vi "Periodic Tasks.vi"(8 "error in":errorcluster) -> ()   [LabVIEW 2017]
doc: "This VI runs in parallel to other robot code. It can contain as many user-defined periodic loops as you need. These can carry out PID or other sorts of timed response."
uses:
  <vilib>/Rock Robotics/Network Tables/NT Write Number.vi
  <vilib>/Rock Robotics/Network Tables/NT Write Boolean.vi
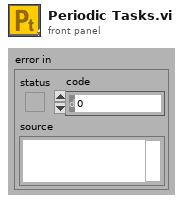
[diagram p1: front panel]
types:
  T1 = typedef "WPI_AnalogChannelDevRef.ctl" = cluster{"DevStatus":errorcluster, "Analog Channel":T2}
  T2 = typedef "FPGA_AIChannel.ctl" = enum8{"AI 0", "AI 1", "AI 2", "AI 3", "AI MXP 0", "AI MXP 1", "AI MXP 2", "AI MXP 3", "Invalid"}
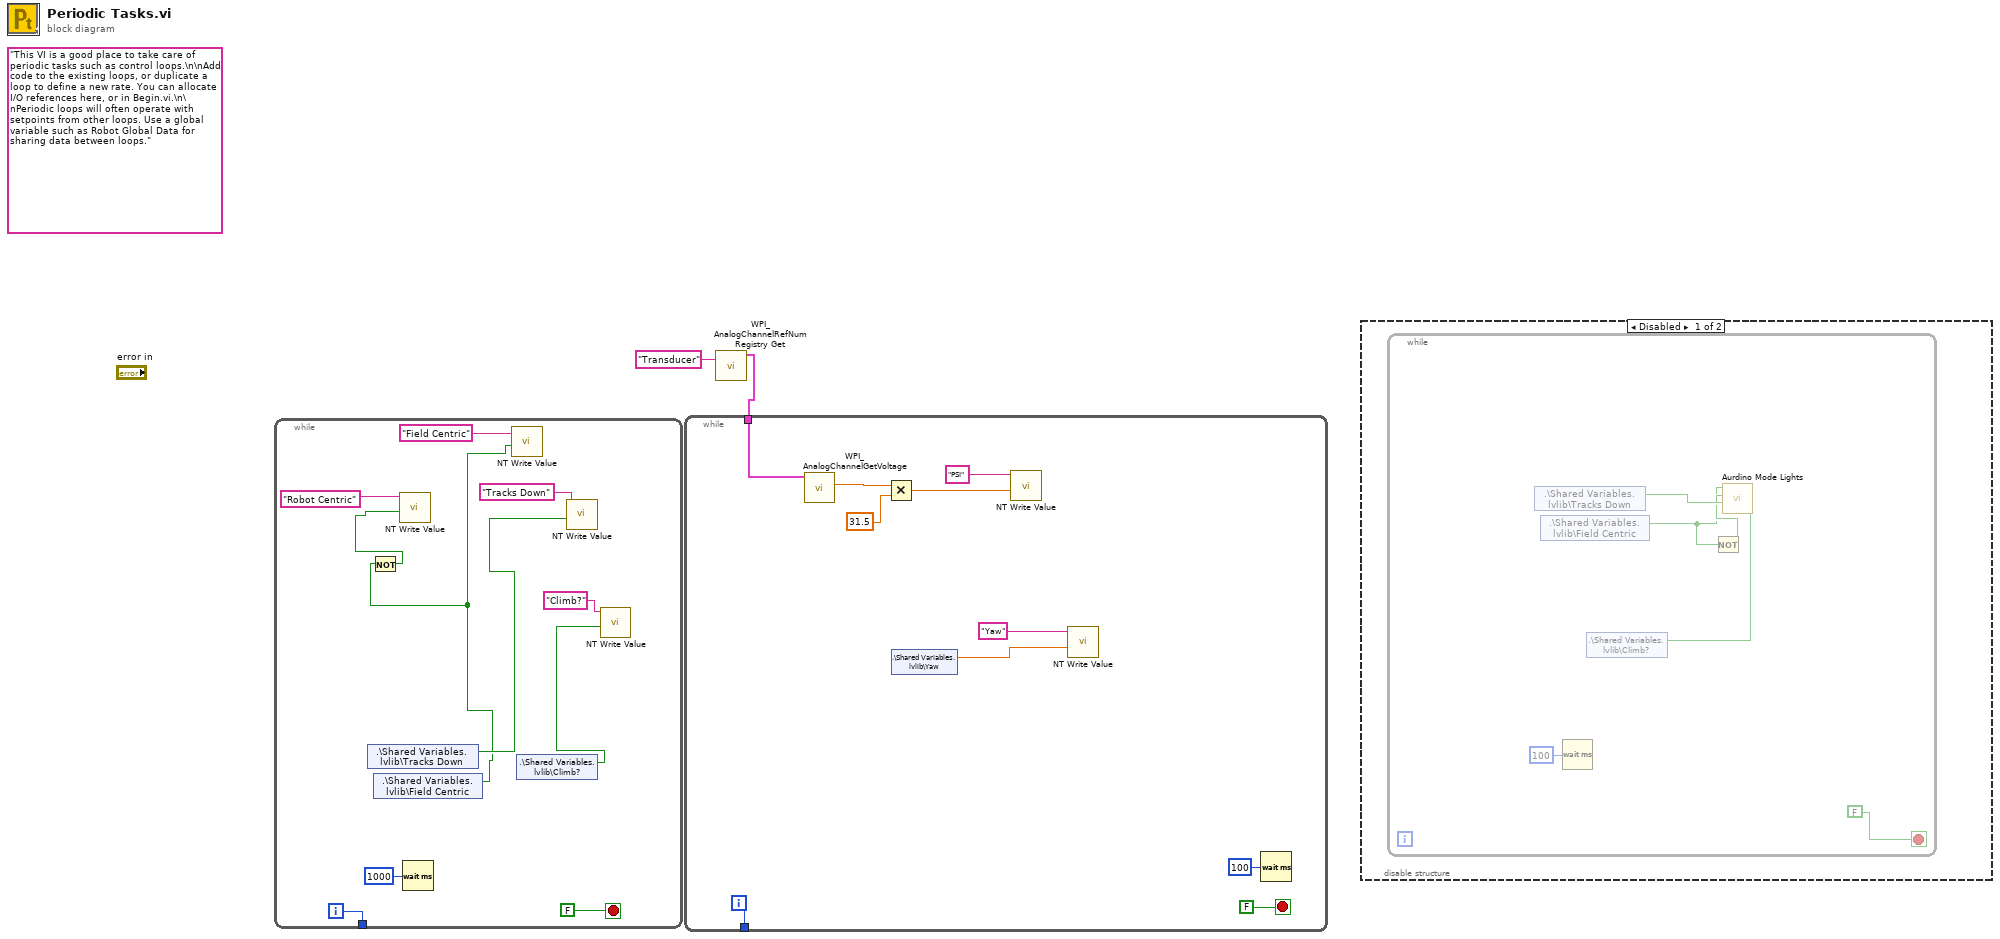
[diagram p0: block diagram]
diagram:
  (unwired) "This VI is a good place to take care of periodic tasks such as control loops.\n\nAdd code to the existing loops, or duplicate a loop to define a new rate. You can allocate I/O references here, or in Begin.vi.\n\nPeriodic loops will often operate with setpoints from other loops. Use a global variable such as Robot Global Data for sharing data between loops."
  n1 = while {
    tunnel: [w12] -> _
    i -> [w12]
    stop <- FALSE stop-if-true
    n2 = shared-variable ".\\Shared Variables.lvlib\\Tracks Down"() -> (w6:bool)  [unwired: 1 in, 1 out]
    n3 = shared-variable ".\\Shared Variables.lvlib\\Field Centric"() -> (w5:bool)  [unwired: 1 in, 1 out]
    n4 = Not(x=w5) -> (.not. x?=w7:bool)
    n5 = call-poly <vilib>:"NT Write Value.vi"("Boolean"=w7, "Name"="Robot Centric") -> ()  [unwired: 9 in, 1 out]
    n6 = Wait (ms)(milliseconds to wait=u32 1000) -> ()  [unwired: 1 out]
    n7 = call-poly <vilib>:"NT Write Value.vi"("Boolean"=w5, "Name"="Field Centric") -> ()  [unwired: 9 in, 1 out]
    n8 = shared-variable ".\\Shared Variables.lvlib\\Climb?"() -> (w3:bool)  [unwired: 1 in, 1 out]
    n9 = call-poly <vilib>:"NT Write Value.vi"("Boolean"=w6, "Name"="Tracks Down") -> ()  [unwired: 9 in, 1 out]
    n10 = call-poly <vilib>:"NT Write Value.vi"("Boolean"=w3, "Name"="Climb?") -> ()  [unwired: 9 in, 1 out]
  }
  n11 = call <vilib>:"WPI_AnalogChannelRefNum Registry Get.vi"("refnum name"="Transducer") -> ("AIDeviceRef"=w2:T1)  [unwired: 9 in, 1 out]
  n12 = while {
    tunnel: w2 -> [w21]
    tunnel: [w20] -> _
    i -> [w20]
    stop <- FALSE stop-if-true
    n13 = call <vilib>:"WPI_AnalogChannelGetVoltage.vi"("AIDeviceRef"=w21) -> ("Voltage"=w17:dbl)  [unwired: 8 in, 2 out]
    n14 = Multiply(x=w17, y=31.5) -> (x*y=w16:dbl)
    n15 = shared-variable ".\\Shared Variables.lvlib\\Yaw"() -> (w18:dbl)  [unwired: 1 in, 1 out]
    n16 = call-poly <vilib>:"NT Write Value.vi"("Numeric"=w16, "Name"="PSI") -> ()  [unwired: 9 in, 1 out]
    n17 = call-poly <vilib>:"NT Write Value.vi"("Numeric"=w18, "Name"="Yaw") -> ()  [unwired: 9 in, 1 out]
    n18 = Wait (ms)(milliseconds to wait=u32 100) -> ()  [unwired: 1 out]
  }
  n19 = disable-structure shown="Disabled" {
    frame Disabled {
      n20 = while {
        stop <- FALSE stop-if-true
        n21 = shared-variable ".\\Shared Variables.lvlib\\Tracks Down"() -> (w27:bool)  [unwired: 1 in, 1 out]
        n22 = shared-variable ".\\Shared Variables.lvlib\\Field Centric"() -> (w25:bool)  [unwired: 1 in, 1 out]
        n23 = Wait (ms)(milliseconds to wait=u32 100) -> ()  [unwired: 1 out]
        n24 = shared-variable ".\\Shared Variables.lvlib\\Climb?"() -> (w24:bool)  [unwired: 1 in, 1 out]
        n25 = Not(x=w25) -> (.not. x?=w26:bool)
        n26 = call "Aurdino Mode Lights.vi"("Climb"=w24, "Tracks Down"=w27, "Robot Centric"=w26, "Field Centric"=w25) -> ()  [unwired: 6 in]
      }
    }
    frame Enabled {
    }
  }
